vi "WriteShell.vi"(8 "error in (no error)":errorcluster, 10 "Shell":refnum<class "zmq_socket.lvclass">, 11 "object in":refnum<class "JuPyter_Client.lvclass">) -> (0 "error out":errorcluster, 3 "object out":refnum<class "JuPyter_Client.lvclass">)   [LabVIEW 2018, in "JuPyter_Client.lvclass"]
uses:
  JuPyter_Client.lvclass
  <vilib>/addons/zeromq/zmq_socket.lvclass
  JuPyter_Client.lvclass/JuPyter_Client.ctl
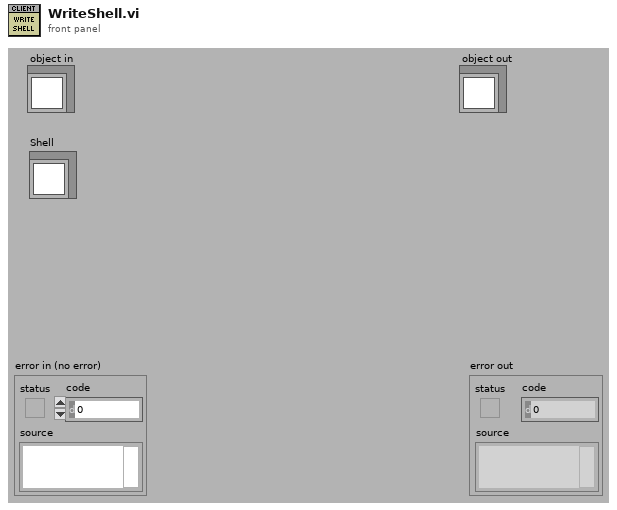
[diagram p1: front panel]
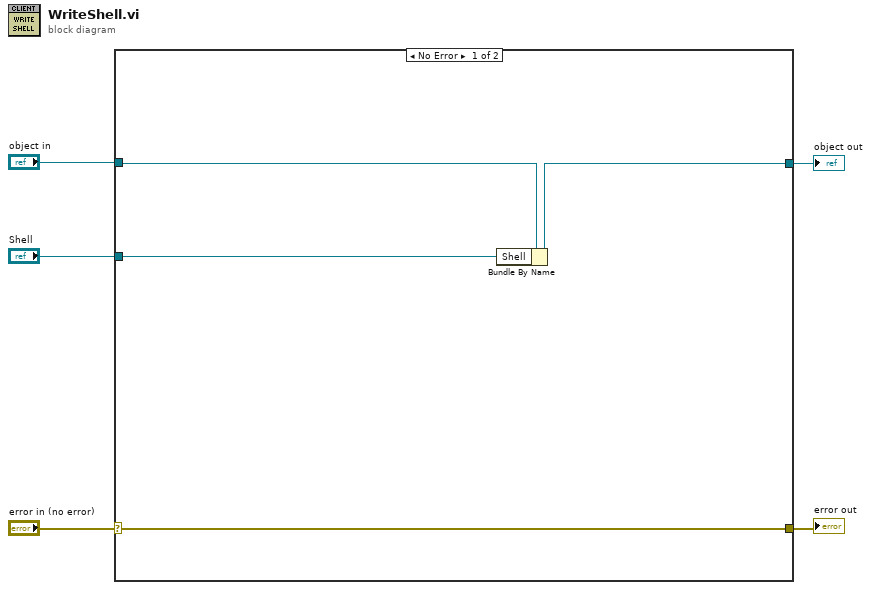
[diagram p0: block diagram]
diagram:
  n1 = case shown="No Error" "error in (no error)" {
    selector: "error in (no error)" -> [w8 w11]
    tunnel: [w8 w11] -> w4
    tunnel: [w6 w10] -> w2
    tunnel: "object in" -> [w7 w10]
    tunnel: "Shell" -> [w9 _]
    frame No Error {
      n2 = Bundle By Name(cluster=w7, "Shell"=w9) -> (w6:refnum<class "JuPyter_Client.lvclass">)
    }
    frame Error {
    }
  }
  "error out" <- w4
  "object out" <- w2
